vi "Read Wave1.vi"(7 "error in":errorcluster, 8 "Wave Offset Input":i32[](array[numeric]), 9 "Iteration of Loop":i32, 10 "refnum":refnum<file>) -> (0 "error out":errorcluster, 1 "Wave Offset":i32[](array[numeric]), 2 "output cluster":T1, 3 "refnum out":refnum<file>)   [LabVIEW 2014]
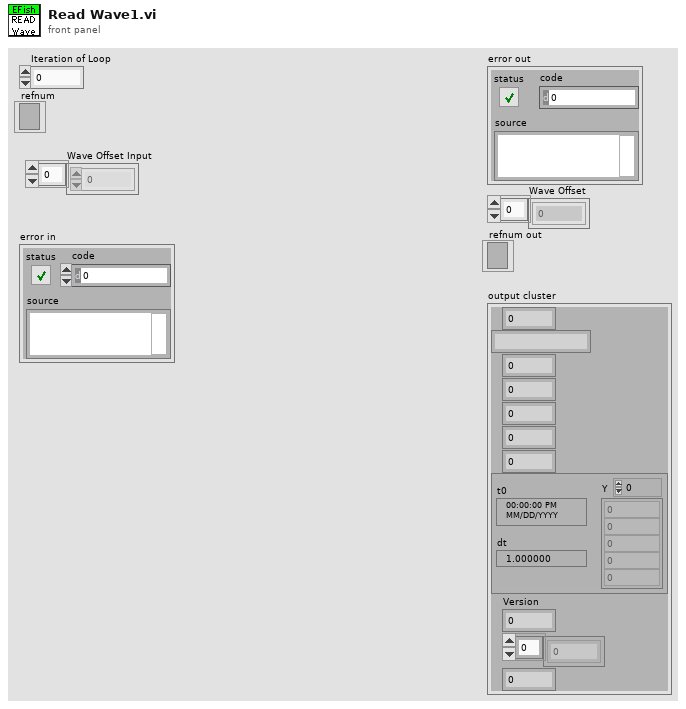
[diagram p1: front panel]
types:
  T1 = cluster{u8, string, i8, i8, i8, u32, u32, "Waveform":waveform(i16), "Version":i32, sgl[], sgl}
  T2 = cluster{u8, string, i8, i8, i8, u32, u32, waveform(i16), "Version":i32, sgl[], sgl}
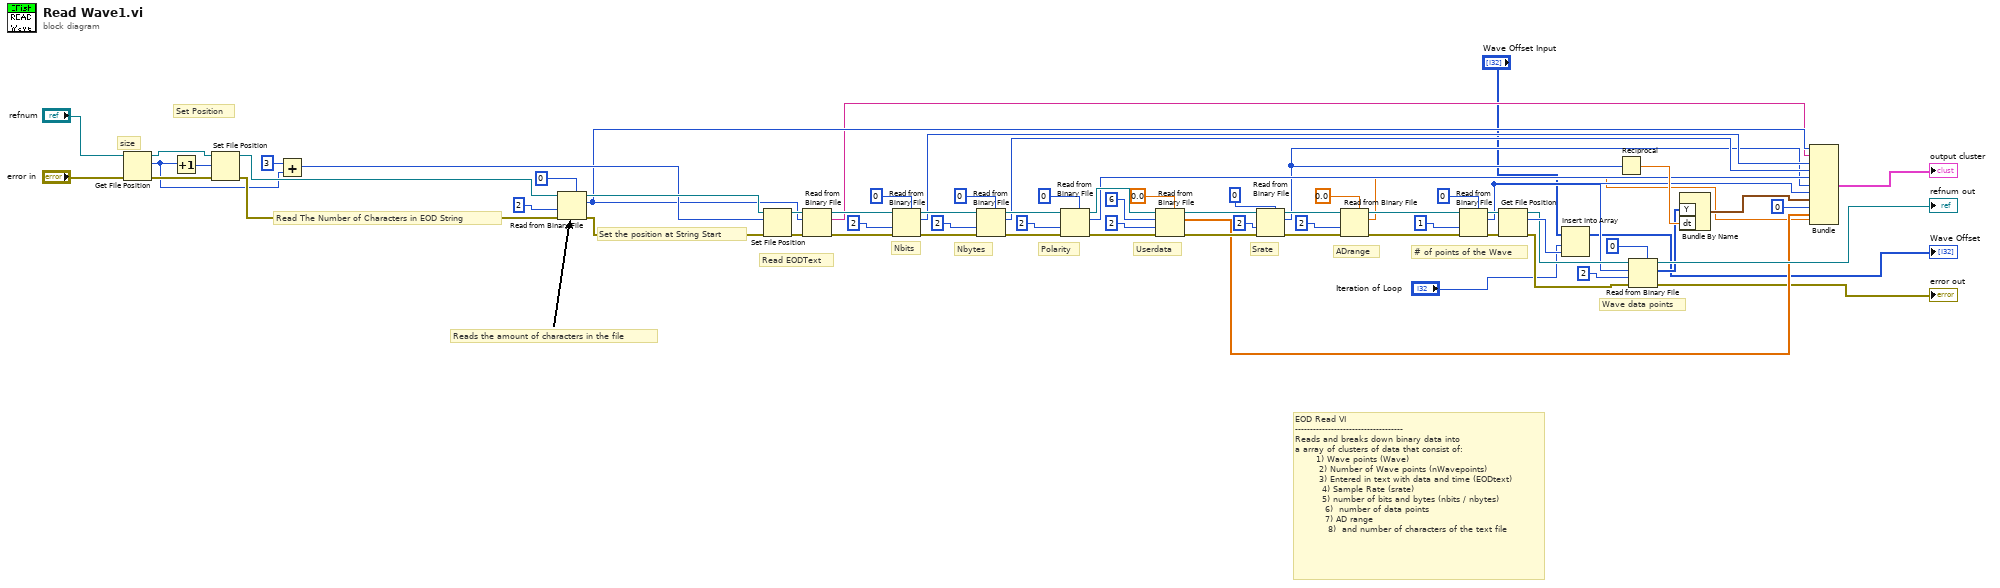
[diagram p0: block diagram]
diagram:
  # "EOD Read VI\n------------------------------------\nReads and breaks down binary data into\na array of clusters of data that consist of:\n       1) Wave points (Wave)\n        2) Number of Wave points (nWavepoints)\n        3) Entered in text with data and time (EODtext)\n         4) Sample Rate (srate) \n         5) number of bits and bytes (nbits / nbytes)\n          6)  number of data points\n          7) AD range\n           8)  and number of characters of the text file"
  # "ADrange"
  # "Nbits"
  # "Reads the amount of characters in the file"
  # "size"
  # "# of points of the Wave"
  # "Wave data points"
  # "Srate"
  # "Userdata"
  # "Polarity"
  # "Nbytes"
  # "Read EODText"
  # "Set the position at String Start"
  # "Read The Number of Characters in EOD String"
  # "Set Position"
  n1 = Get File Position(4:"error in", 7:"refnum") -> (0:w31:errorcluster, 2:w19:i64, 3:w32:refnum<file>)
  n2 = Increment(x=w19) -> (x+1=w28:i64)
  n3 = Set File Position(offset (in bytes) (0)=w28, refnum=w32, error in=w31) -> (refnum out=w70:refnum<file>, error out=w42:errorcluster)  [unwired: 1 in]
  n4 = Add(x=3, y=w19) -> (x+y=w30:i64)
  n5 = Read from Binary File(5:u8 0, 8:w42, 9:2, 11:w70) -> (0:w41:errorcluster, 2:w18:u8, 3:w69:refnum<file>)  [unwired: 2 in, 1 out]
  n6 = Set File Position(offset (in bytes) (0)=w30, refnum=w69, error in=w41) -> (refnum out=w68:refnum<file>, error out=w40:errorcluster)  [unwired: 1 in]
  n7 = Read from Binary File(8:w40, 10:w18, 11:w68) -> (0:w39:errorcluster, 2:w17:string, 3:w67:refnum<file>)  [unwired: 3 in, 1 out]
  n8 = Read from Binary File(5:i8 0, 8:w39, 9:2, 11:w67) -> (0:w38:errorcluster, 2:w16:i8, 3:w44:refnum<file>)  [unwired: 2 in, 1 out]
  n9 = Read from Binary File(5:i8 0, 8:w38, 9:2, 11:w44) -> (0:w37:errorcluster, 2:w15:i8, 3:w45:refnum<file>)  [unwired: 2 in, 1 out]
  n10 = Read from Binary File(5:i8 0, 8:w37, 9:2, 11:w45) -> (0:w36:errorcluster, 2:w14:i8, 3:w43:refnum<file>)  [unwired: 2 in, 1 out]
  n11 = Read from Binary File(5:sgl 0.0, 8:w36, 9:2, 10:6, 11:w43) -> (0:w35:errorcluster, 2:w9:sgl[], 3:w64:refnum<file>)  [unwired: 1 in, 1 out]
  n12 = Read from Binary File(5:u32 0, 8:w35, 9:2, 11:w64) -> (0:w34:errorcluster, 2:w13:u32, 3:w56:refnum<file>)  [unwired: 2 in, 1 out]
  n13 = Read from Binary File(5:sgl 0.0, 8:w34, 9:2, 11:w56) -> (0:w33:errorcluster, 2:w8:sgl, 3:w51:refnum<file>)  [unwired: 2 in, 1 out]
  n14 = Read from Binary File(5:u32 0, 8:w33, 9:1, 11:w51) -> (0:w23:errorcluster, 2:w12:u32, 3:w25:refnum<file>)  [unwired: 2 in, 1 out]
  n15 = Get File Position(4:w23, 7:w25) -> (0:w22:errorcluster, 2:w26:i64, 3:w24:refnum<file>)
  n16 = Insert Into Array(array="Wave Offset Input", index="Iteration of Loop", new element=w26) -> (→"Wave Offset":i32[])
  n17 = Reciprocal(x=w13) -> (1/x=w21:dbl)
  n18 = Read from Binary File(5:i16 0, 8:w22, 9:2, 10:w12, 11:w24) -> (0:→"error out":errorcluster, 2:w20:i16[], 3:→"refnum out":refnum<file>)  [unwired: 1 in, 1 out]
  n19 = Bundle By Name("Y"=w20, "dt"=w21) -> (w11:waveform(i16))  [unwired: 1 in]
  n20 = Bundle(w18, w17, w16, w15, w14, w13, w12, w11, "Version"=0, w9, w8) -> (→"output cluster":T2)  [unwired: 1 in]
